vi "testing odor and manifold config dialog.vi"() -> ()   [LabVIEW 2021]
uses:
  type-defs/odor and manifold config cluster (type def).ctl
  type-defs/manifold configuration cluster array (type def).ctl
  type-defs/manifold configuration cluster (type def).ctl
  type-defs/manifold selection.ctl
  type-defs/single port single odor cluster.ctl
  type-defs/port number (type def).ctl
  type-defs/odor selection (type def).ctl
  type-defs/odor color (type def).ctl
  type-defs/odor description array (type def).ctl
  type-defs/odor info cluster (type def).ctl
  <vilib>/ErrorRing/Error Ring.xnode
panel:
  in  "Stop":bool
  out "odor & manifold config cluster":T1
  in  "configure odor-manifold":bool
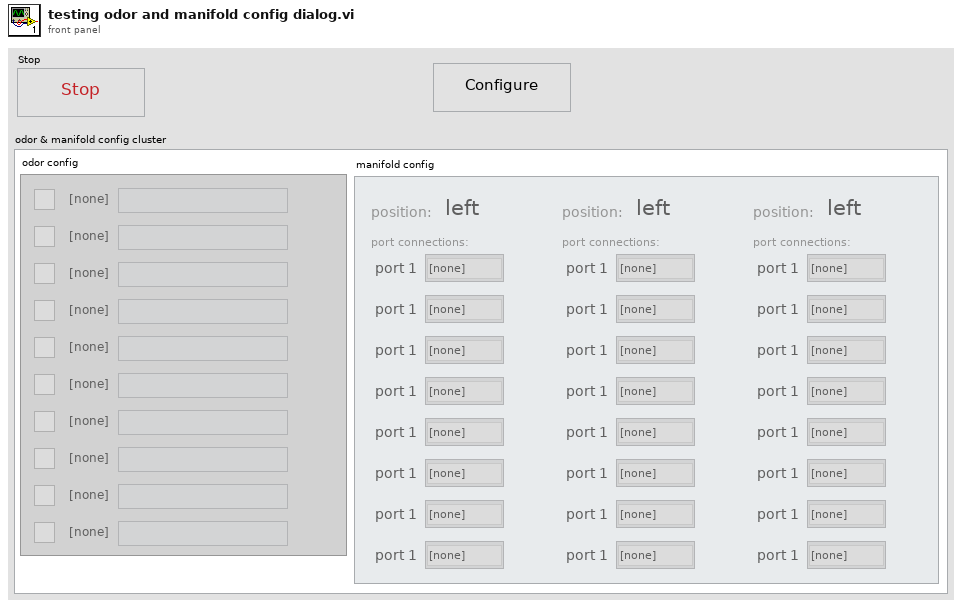
[diagram p1: front panel]
types:
  T1 = typedef "odor and manifold config cluster (type def).ctl" = cluster{"manifold config":T2, "odor config":T9}
  T2 = typedef "manifold configuration cluster array (type def).ctl" = T3[]
  T3 = typedef "manifold configuration cluster (type def).ctl" = cluster{"position:":T4, "port connections:":T5[]}
  T4 = typedef "manifold selection.ctl" = enum16{"left", "middle", "right"}
  T5 = typedef "single port single odor cluster.ctl" = cluster{"port number":T6, "connected odor":T7, "error":bool, "odor color":T8}
  T6 = typedef "port number (type def).ctl" = enum16{"port 1", "port 2", "port 3", "port 4", "port 5", "port 6", "port 7", "port 8"}
  T7 = typedef "odor selection (type def).ctl" = enum16{"[none]", "odor 1", "odor 2", "odor 3", "odor 4", "odor 5", "odor 6", "odor 7", "odor 8", "odor 9", "odor 10"}
  T8 = typedef "odor color (type def).ctl" = u16
  T9 = typedef "odor description array (type def).ctl" = T10[]
  T10 = typedef "odor info cluster (type def).ctl" = cluster{"odor channel":T7, "odor description":string, "odor color":T8, "odor channel active":bool}
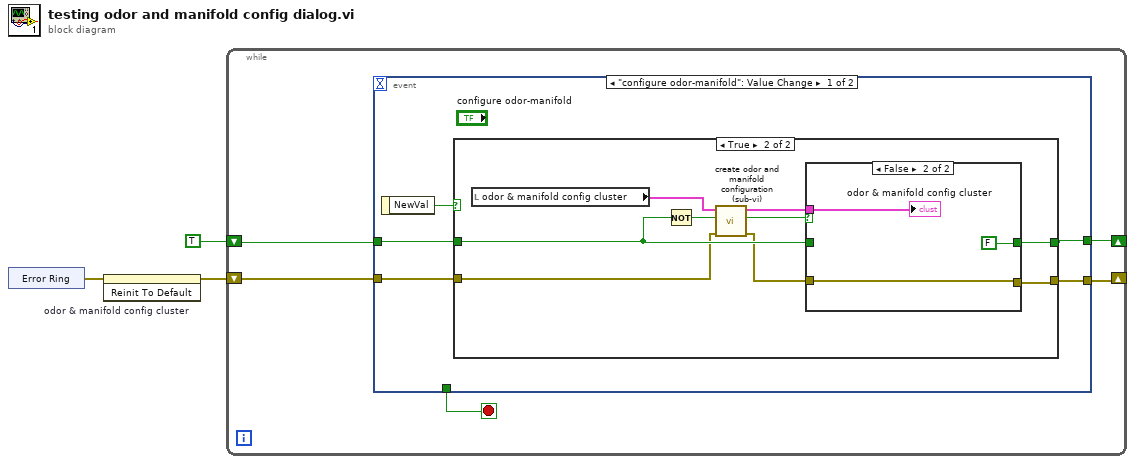
[diagram p0: block diagram]
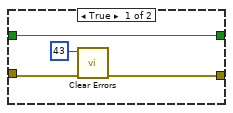
[diagram p3: hidden frame]
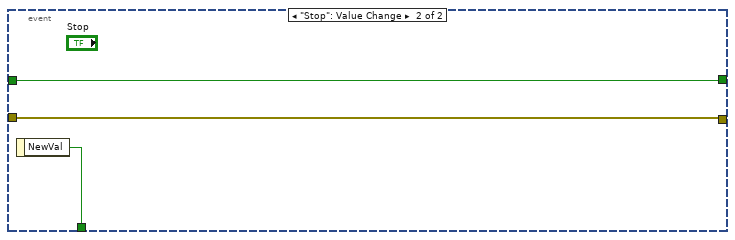
[diagram p4: hidden frame]
diagram:
  n1 = xnode "Error Ring"() -> ("error out"=w2:errorcluster)
  n2 = invoke on="odor & manifold config cluster" class="Clust (strict)" method="Reinit To Default"(error in=w2) -> (error out=w1:errorcluster)  [unwired: 2 in, 2 out]
  n3 = while {
    shift-right: [w7] -> _
    shift-left: TRUE -> [w8]
    shift-right: [w4] -> _
    shift-left: w1 -> [w5]
    stop <- w6 stop-if-true
    n4 = event shown="[0] \"configure odor-manifold\": Value Change" {
      selector: _ -> [_ _]
      dyn-events: _ -> [_ _]
      timeout: _ -> [_ _]
      tunnel: w8 -> [w12 w33]
      tunnel: [w11 w33] -> w7
      tunnel: [_ w34] -> w6
      tunnel: w5 -> [w10 w32]
      tunnel: [w9 w32] -> w4
      event "configure odor-manifold": Value Change {
        n5 = event-data() -> ("NewVal"=w13:bool)  [unwired: 1 in]
        n6 = case shown="True" w13 {
          tunnel: w12 -> [w15 w20]
          tunnel: [w15 w19] -> w11
          tunnel: w10 -> [w14 w18]
          tunnel: [w14 w16] -> w9
          frame False {
          }
          frame True {
            n7 = local read "odor & manifold config cluster"() -> (w22:T1)
            n8 = Not(x=w20) -> (.not. x?=w21:bool)
            n9 = call "create odor and manifold configuration (sub-vi).vi"("error in (no error)"=w18, "use initial config? (F)"=w21, "initial odor and manifold config (none)"=w22) -> ("error out"=w17:errorcluster, "operation failed?"=w23:bool, "odor and manifold config out"=w24:T1)  [unwired: 6 in]
            n10 = case shown="False" w23 {
              tunnel: w24 -> [_ w31]
              tunnel: w20 -> [w28 _]
              tunnel: [w28 FALSE] -> w19
              tunnel: w17 -> [w27 w29]
              tunnel: [w26 w29] -> w16
              frame True {
                n11 = call <vilib>:"Clear Errors.vi"("error in (no error)"=w27, "specific error code to clear (0: all)"=43) -> ("error out"=w26:errorcluster)  [unwired: 4 in, 1 out]
              }
              frame False {
                "odor & manifold config cluster" <- w31
              }
            }
          }
        }
      }
      event "Stop": Value Change {
        n12 = event-data() -> ("NewVal"=w34:bool)  [unwired: 1 in]
      }
    }
  }
